vi "Read Index.vi"(8 "error in (no error)":errorcluster, 11 "GenericDevice in":refnum<class "GenericDevice.lvclass">) -> (0 "error out":errorcluster, 2 "Index":i32, 3 "GenericDevice out":refnum<class "GenericDevice.lvclass">)   [LabVIEW 2020, in "horiba.lvlib" / "GenericDevice.lvclass"]
doc: "Accessor VI for this class property."
uses:
  GenericDevice.lvclass
  GenericDevice.lvclass/GenericDevice.ctl
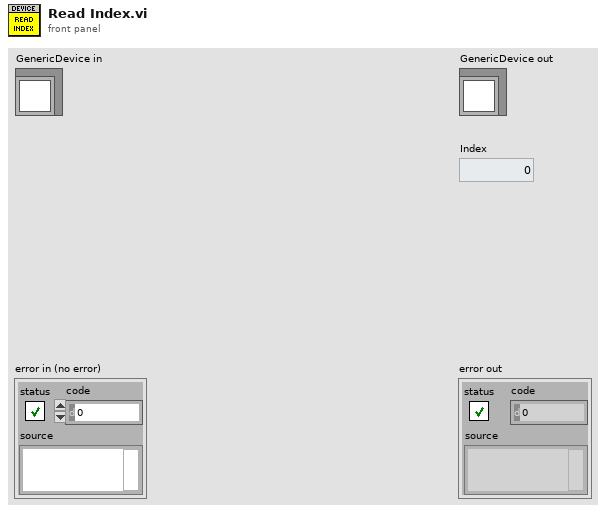
[diagram p1: front panel]
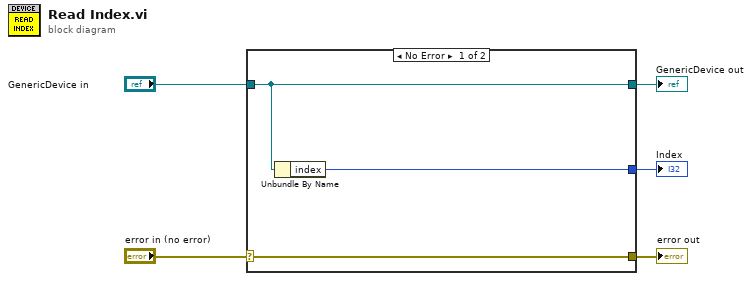
[diagram p0: block diagram]
diagram:
  n1 = case shown="No Error" "error in (no error)" {
    selector: "error in (no error)" -> [w8 w9]
    tunnel: [w8 w9] -> w4
    tunnel: [w7 w10] -> w2
    tunnel: "GenericDevice in" -> [w7 w10]
    tunnel: [w6 _] -> w1
    frame No Error {
      n2 = Unbundle By Name(w7) -> ("index"=w6:i32)
    }
    frame Error {
    }
  }
  "error out" <- w4
  "GenericDevice out" <- w2
  "Index" <- w1
